vi "PJT_06.vi"() -> ()   [LabVIEW 2019]
panel:
  out "XY 그래프":cluster{dbl[], dbl[]}(graph)
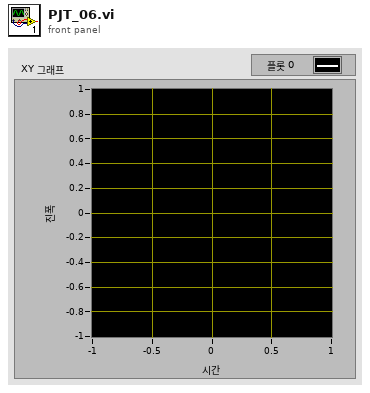
[diagram p1: front panel]
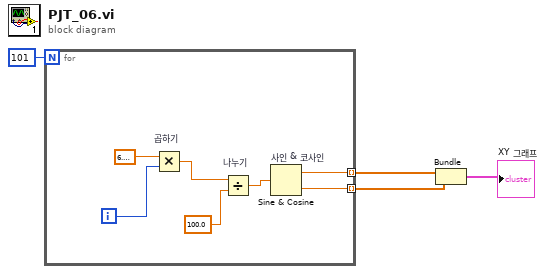
[diagram p0: block diagram]
diagram:
  n1 = for {
    N: 101 -> [_]
    tunnel: [w6] -> w3 mode=indexing
    tunnel: [w5] -> w2 mode=indexing
    i -> [w8]
    n2 = Multiply "곱하기"(x=6.283185307179586, y=w8) -> (x*y=w11:dbl)
    n3 = Divide "나누기"(x=w11, y=100.0) -> (x/y=w9:dbl)
    n4 = Sine & Cosine "사인 & 코사인"(0:w9) -> (1:w6:dbl, 2:w5:dbl)
  }
  n5 = Bundle(w3, w2) -> (→"XY 그래프":cluster{dbl[], dbl[]})  [unwired: 1 in]
